vi "Init.vi"(8 "error in":errorcluster, 10 "OD Entry":refnum<class "OD Entry.lvclass">) -> (0 "error out":errorcluster, 3 "Transmit PDO out":refnum<class "PDO Communication Parameter.lvclass">)   [LabVIEW 2024, in "PDO Grid.lvlib" / "PDO Communication Parameter.lvclass"]
uses:
  PDO Communication Parameter.lvclass
  OD Entry/OD Entry.lvclass
  PDO Communication Parameter.lvclass/PDO Communication Parameter.ctl
  Set OD Index.vi
  Set AccessType.vi
  Set Description.vi
  OD Entry/Get AccessType.vi
  OD Entry/Get Description.vi
  Electronic Datasheet.lvlib
  Value/Value.lvclass
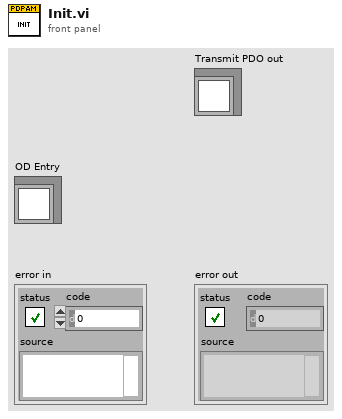
[diagram p1: front panel]
types:
  T1 = typedef "Electronic Datasheet.lvlib/Access Type.ctl" = enum16{"ro", "wo", "rw", "rwr", "rww", "const"}
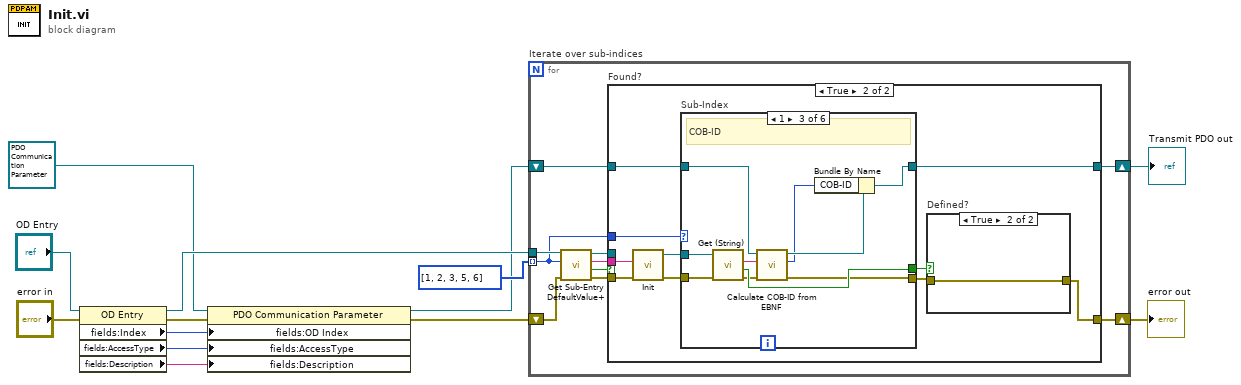
[diagram p0: block diagram]
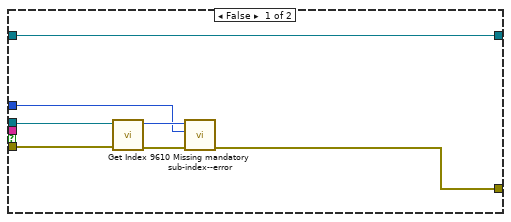
[diagram p2: hidden frame]
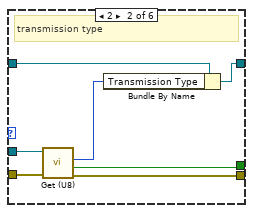
[diagram p4: hidden frame]
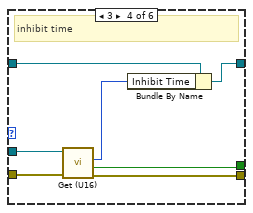
[diagram p5: hidden frame]
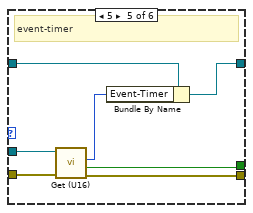
[diagram p6: hidden frame]
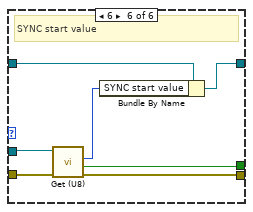
[diagram p7: hidden frame]
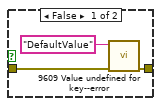
[diagram p8: hidden frame]
diagram:
  n1 = property class="OD Entry"(reference="OD Entry", error in="error in") -> (reference out=w7:refnum<class "OD Entry.lvclass">, error out=w9:errorcluster, "fields:Index"=w3:u16, "fields:AccessType"=w2:T1, "fields:Description"=w1:string)
  n2 = property class="PDO Communication Parameter"(reference=refnum<class "PDO Communication Parameter.lvclass"> refnum ("Transmit PDO in"), error in=w9, "fields:OD Index"=w3, "fields:AccessType"=w2, "fields:Description"=w1) -> (reference out=w4:refnum<class "PDO Communication Parameter.lvclass">, error out=w6:errorcluster)
  n3 = for "Iterate over sub-indices" {
    tunnel: u16[] [1, 2, 3, 5, 6] -> [w18] mode=indexing
    shift-right: [w22] -> w10
    shift-left: w4 -> [w23]
    shift-right: [w21] -> w11
    shift-left: w6 -> [w17]
    tunnel: w7 -> [w20]
    n4 = call "Get Sub-Entry DefaultValue+.vi"("Error In"=w17, "Sub-Index"=w18, "reference in"=w20) -> ("Error Out"=w16:errorcluster, "Found?"=w15:bool, "DefaultValue"=w14:string, "reference out"=w19:refnum<class "OD Entry.lvclass">)  [unwired: 5 in]
    n5 = case "Found?" shown="True" w15 {
      tunnel: w23 -> [w24 w40]
      tunnel: [w24 w39] -> w22
      tunnel: [w25 w32] -> w21
      tunnel: w19 -> [w27 _]
      tunnel: w18 -> [w26 w38]
      tunnel: w16 -> [w28 w37]
      tunnel: w14 -> [_ w31]
      frame False {
        n6 = call "Get Index.vi"("Error In"=w28, "reference in"=w27) -> ("Error Out"=w30:errorcluster, "Index"=w29:u16)  [unwired: 7 in, 1 out]
        n7 = call "9610 Missing mandatory sub-index--error.vi"("error in (no error)"=w30, "Sub-Index"=w26, "Index"=w29) -> ("error out"=w25:errorcluster)  [unwired: 8 in]
      }
      frame True {
        n8 = call "Init.vi"("error in"=w37, "Value"=w31) -> ("error out"=w36:errorcluster, "Value out"=w35:refnum<class "Value.lvclass">)  [unwired: 8 in]
        n9 = case "Sub-Index" shown="1" w38 {
          tunnel: w40 -> [w42 w49 w54 w65 w72 w77]
          tunnel: [w42 w48 w53 w64 w71 w76] -> w39
          tunnel: w36 -> [w41 w46 w56 w61 w70 w79]
          tunnel: w35 -> [_ w45 w58 w62 w69 w74]
          tunnel: [_ w44 w57 w59 w67 w73] -> w34
          tunnel: [w41 w43 w51 w60 w68 w78] -> w33
          frame Default {
            # "can't be reached"
          }
          frame 2 {
            # "transmission type"
            n10 = call "Get (U8).vi"("error in"=w46, "Value in"=w45) -> ("error out"=w43:errorcluster, "Defined?"=w44:bool, "Value"=w47:u8)  [unwired: 6 in, 1 out]
            n11 = Bundle By Name(cluster=w49, "Transmission Type"=w47) -> (w48:refnum<class "PDO Communication Parameter.lvclass">)
          }
          frame 1 {
            # "COB-ID"
            n12 = call "Get (String).vi"("Value in"=w58) -> ("Defined?"=w57:bool, "Value"=w55:string)  [unwired: 8 in, 1 out]
            n13 = call "Calculate COB-ID from EBNF.vi"("error in"=w56, "ENBF"=w55, "Transmit PDO in"=w54) -> ("error out"=w51:errorcluster, "COB-ID"=w50:u32, "Transmit PDO out"=w52:refnum<class "PDO Communication Parameter.lvclass">)  [unwired: 6 in]
            n14 = Bundle By Name(cluster=w52, "COB-ID"=w50) -> (w53:refnum<class "PDO Communication Parameter.lvclass">)
          }
          frame 3 {
            # "inhibit time"
            n15 = call "Get (U16).vi"("error in"=w61, "Value in"=w62) -> ("error out"=w60:errorcluster, "Defined?"=w59:bool, "Value"=w63:u16)  [unwired: 6 in, 1 out]
            n16 = Bundle By Name(cluster=w65, "Inhibit Time"=w63) -> (w64:refnum<class "PDO Communication Parameter.lvclass">)
          }
          frame 5 {
            # "event-timer"
            n17 = call "Get (U16).vi"("error in"=w70, "Value in"=w69) -> ("error out"=w68:errorcluster, "Defined?"=w67:bool, "Value"=w66:u16)  [unwired: 6 in, 1 out]
            n18 = Bundle By Name(cluster=w72, "Event-Timer"=w66) -> (w71:refnum<class "PDO Communication Parameter.lvclass">)
          }
          frame 6 {
            # "SYNC start value"
            n19 = call "Get (U8).vi"("error in"=w79, "Value in"=w74) -> ("error out"=w78:errorcluster, "Defined?"=w73:bool, "Value"=w75:u8)  [unwired: 6 in, 1 out]
            n20 = Bundle By Name(cluster=w77, "SYNC start value"=w75) -> (w76:refnum<class "PDO Communication Parameter.lvclass">)
          }
        }
        n21 = case "Defined?" shown="True" w34 {
          tunnel: w33 -> [w82 w83]
          tunnel: [w81 w83] -> w32
          frame False {
            n22 = call "9609 Value undefined for key--error.vi"("error in"=w82, "key"="DefaultValue") -> ("error out"=w81:errorcluster)  [unwired: 9 in]
          }
          frame True {
          }
        }
      }
    }
  }
  "Transmit PDO out" <- w10
  "error out" <- w11
